vi "befor_ChkSum.vi"(11 "ToolString Input":string="$AGENT,53,VS-62U009+VS-69W014*71") -> (2 "ToolString Output":string, 3 "Array":string[](array[string]))   [LabVIEW 2019]
panel:
  out "ToolString Input 2":string
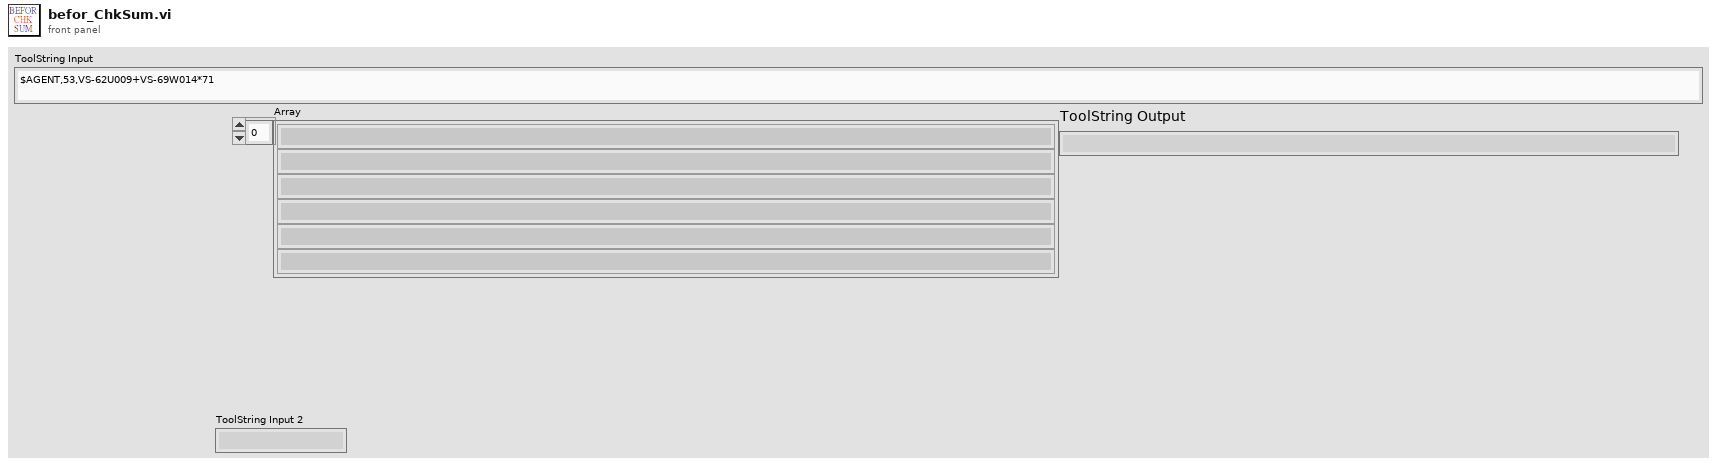
[diagram p1: front panel]
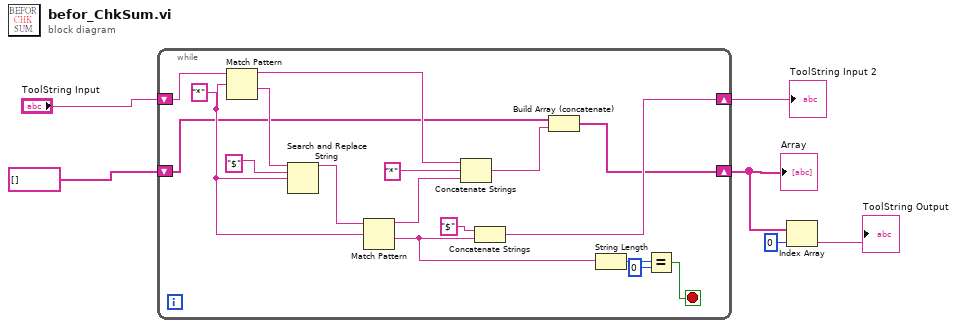
[diagram p0: block diagram]
diagram:
  n1 = while {
    shift-right: [w14] -> w4
    shift-left: "ToolString Input" -> [w15]
    shift-right: [w11] -> w3
    shift-left: string[] [] -> [w13]
    stop <- w7 stop-if-true
    w21 = "*" ("regular expression")
    n2 = Match Pattern(string=w15, regular expression=w21) -> (before substring=w19:string, after substring=w20:string)  [unwired: 1 in, 2 out]
    n3 = Search and Replace String(input string=w20, search string="$" ("regular expression"), replace string=w21) -> (result string=w22:string)  [unwired: 5 in, 3 out]
    n4 = Match Pattern(string=w22, regular expression=w21) -> (before substring=w17:string, after substring=w8:string)  [unwired: 1 in, 2 out]
    n5 = Concatenate Strings(w19, "*" ("string"), w17) -> (w12:string)
    n6 = Concatenate Strings("$" ("regular expression"), w8) -> (w14:string)
    n7 = Build Array (concatenate)(w13, w12) -> (w11:string[])
    n8 = String Length(string=w8) -> (length=w10:i32)
    n9 = Equal?(x=w10, y=0) -> (x = y?=w7:bool)
  }
  "Array" <- w3
  "ToolString Input 2" <- w4
  n10 = Index Array(array=w3, index=0) -> (element=→"ToolString Output":string)
